vi "set_params.vi"(8 "error in (no error)":errorcluster, 11 "ibsen in":refnum<class "ibsen.lvclass">) -> (0 "error out":errorcluster, 3 "ibsen out":refnum<class "ibsen.lvclass">)   [LabVIEW 2019, in "ibsen.lvlib" / "ibsen.lvclass"]
uses:
  ibsen.lvclass
  _camera/_camera.lvlibp/_cameraClass/_camera.lvclass
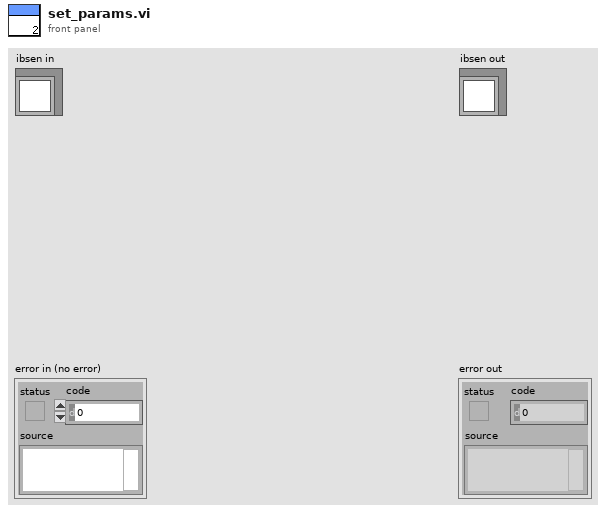
[diagram p1: front panel]
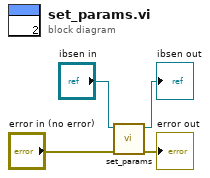
[diagram p0: block diagram]
diagram:
  n1 = call-parent "set_params.vi"("error in (no error)"="error in (no error)", "_camera in"="ibsen in") -> ("error out"=→"error out":errorcluster, "_camera out"=→"ibsen out":refnum<class "ibsen.lvclass">)  [unwired: 8 in]
